vi "Clear.vi"(8 "error in (no error)":errorcluster, 11 "DAQmx in":refnum<class "DAQmx.lvclass">) -> (0 "error out":errorcluster, 3 "DAQmx out":refnum<class "DAQmx.lvclass">)   [LabVIEW 2019, in "DAQmx.lvclass"]
uses:
  DAQmx.lvclass
  DAQmx.lvclass/DAQmx.ctl
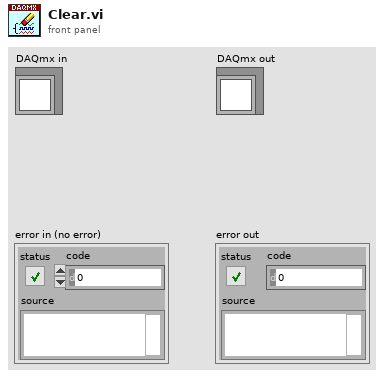
[diagram p1: front panel]
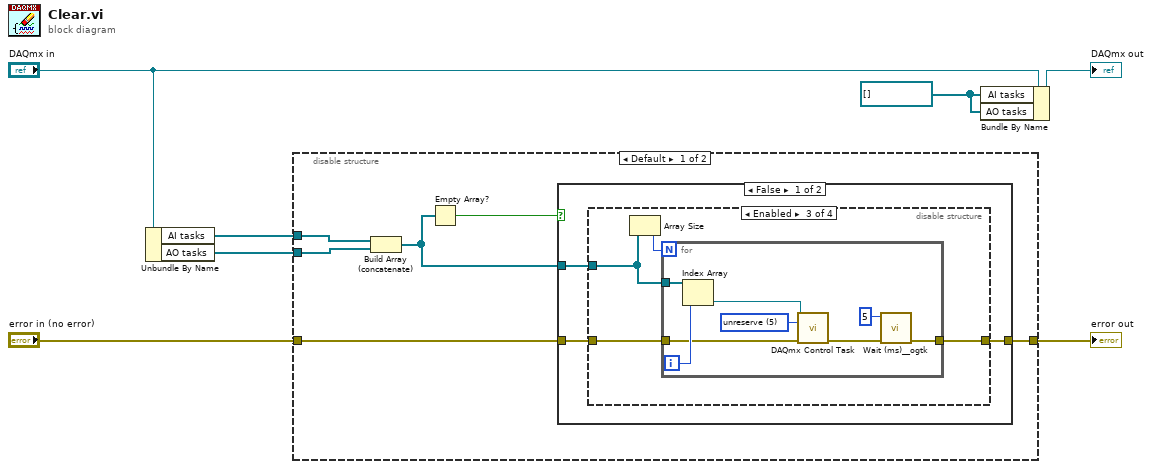
[diagram p0: block diagram]
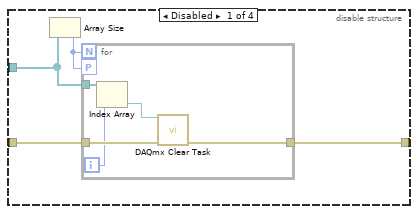
[diagram p2: hidden frame]
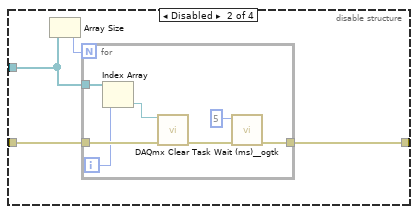
[diagram p3: hidden frame]
diagram:
  w1 = refnum<k21>[] [] ("AI task")
  n1 = Unbundle By Name("DAQmx in") -> ("AI tasks"=w4:refnum<k21>[], "AO tasks"=w5:refnum<k21>[])
  n2 = disable-structure shown="Default" {
    disable-tunnel: "error in (no error)" -> [w8 _]
    disable-tunnel: [w11 _] -> w6
    disable-tunnel: w5 -> [w12 _]
    disable-tunnel: w4 -> [w13 _]
    frame condition #0 (active) {
      n3 = Build Array (concatenate)(w13, w12) -> (w9:refnum<k21>[])
      n4 = Empty Array?(array=w9) -> (empty?=w10:bool)
      n5 = case shown="False" w10 {
        tunnel: w8 -> [w15 w49]
        tunnel: w9 -> [w14 _]
        tunnel: [w16 w49] -> w11
        frame False {
          n6 = disable-structure shown="Enabled" {
            disable-tunnel: [w20 w29 w40 _] -> w16
            disable-tunnel: w15 -> [w19 w28 w39 _]
            disable-tunnel: w14 -> [w17 w26 w37 _]
            frame Disabled {
              n7 = Array Size(array=w17) -> (size(s)=w18:i32)
              n8 = for {
                N: w18 -> [_]
                tunnel: w17 -> [w23]
                tunnel: w19 -> [w25]
                tunnel: [w22] -> w20
                workers-P: w18 -> [_]
                i -> [w24]
                n9 = Index Array(array=w23, index=w24) -> (element=w21:refnum<k21>)
                n10 = call <vilib>:"DAQmx Clear Task.vi"("task in"=w21, "error in"=w25) -> ("error out"=w22:errorcluster)  [unwired: 13 in]
              }
            }
            frame Disabled {
              n11 = Array Size(array=w26) -> (size(s)=w27:i32)
              n12 = for {
                N: w27 -> [_]
                tunnel: w26 -> [w34]
                tunnel: w28 -> [w36]
                tunnel: [w31] -> w29
                i -> [w35]
                n13 = Index Array(array=w34, index=w35) -> (element=w32:refnum<k21>)
                n14 = call <vilib>:"DAQmx Clear Task.vi"("task in"=w32, "error in"=w36) -> ("error out"=w33:errorcluster)  [unwired: 13 in]
                n15 = call <userlib>:"Wait (ms)__ogtk.vi"("error in (no error)"=w33, "milliseconds to wait"=u32 5) -> ("error out"=w31:errorcluster)  [unwired: 8 in, 1 out]
              }
            }
            frame Enabled {
              n16 = Array Size(array=w37) -> (size(s)=w38:i32)
              n17 = for {
                N: w38 -> [_]
                tunnel: w37 -> [w47]
                tunnel: w39 -> [w42]
                tunnel: [w46] -> w40
                i -> [w48]
                w44 = 5 items=["verify"=2, "reserve"=4, "commit"=3, "unreserve"=5, "abort"=6] ("action")
                n18 = Index Array(array=w47, index=w48) -> (element=w43:refnum<k21>)
                n19 = call <vilib>:"DAQmx Control Task.vi"("task/channels in"=w43, "action"=w44, "error in"=w42) -> ("error out"=w41:errorcluster)  [unwired: 11 in, 1 out]
                n20 = call <userlib>:"Wait (ms)__ogtk.vi"("error in (no error)"=w41, "milliseconds to wait"=u32 5) -> ("error out"=w46:errorcluster)  [unwired: 8 in, 1 out]
              }
            }
            frame Disabled {
            }
          }
        }
        frame True {
        }
      }
    }
    frame condition #1 {
    }
  }
  "error out" <- w6
  n21 = Bundle By Name(cluster="DAQmx in", "AI tasks"=w1, "AO tasks"=w1) -> (→"DAQmx out":refnum<class "DAQmx.lvclass">)
